vi "Run.vi"(8 "error in (no error)":errorcluster, 11 "LINX in":refnum<class "LINX.lvclass">) -> (0 "error out":errorcluster, 3 "LINX out":refnum<class "LINX.lvclass">)   [LabVIEW 2019, in "LINX.lvlib" / "LINX.lvclass"]
doc: "<b>Execution System:</b> Data Acquisition"
uses:
  LINX.lvclass
  <vilib>/MakerHub/LINX/Public/Peripherals/Analog/Analog Read N Chans.vi
  <vilib>/MakerHub/LINX/Public/Peripherals/Digital/Digital Read N Chans.vi
  <vilib>/MakerHub/LINX/Private/Local IO/LinxAnalogRead.vi
  <vilib>/MakerHub/LINX/Public/Utilities/Check Channel.vi
  <vilib>/MakerHub/LINX/Private/Local IO/LinxDigitalRead.vi
  <vilib>/MakerHub/LINX/Public/Utilities/Open Serial.vi
  <vilib>/MakerHub/LINX/Private/Utilties/Generate Error.vi
  Packed Libraries/Messaging.lvlibp/Send.vi
  Plugin Interfaces/Controller Interface/Controller Interface.lvlibp/Controller Interface Class/Controller Interface.lvclass
  <vilib>/MakerHub/LINX/LMH-LINX.lvlib
  C:/github/dataflowg/dataflow-dj/src/Plugin Interfaces/Controller Interface/Controller Interface.lvlibp/Controller Interface Class/Controller Interface.lvclass
panel:
  out "Error":errorcluster
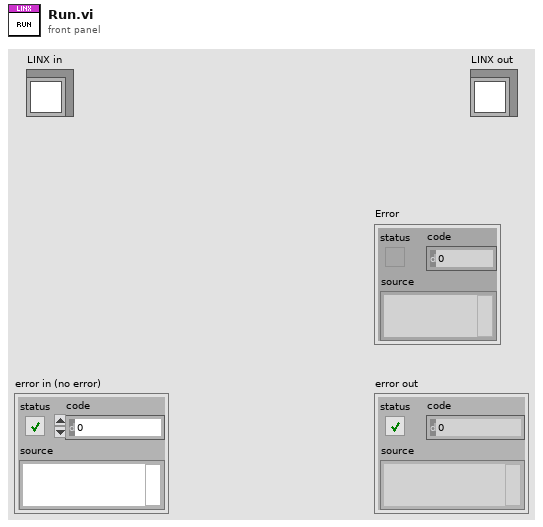
[diagram p1: front panel]
types:
  T1 = typedef "LINX.lvlib/LINX.lvclass/LINX Control Shortcut.ctl" = cluster{"Channel Type":T2, "Channel Number":u8, "Message Queue":string, "Event":string, "Target":string, "Momentary":bool, "Data":variant}
  T2 = typedef "LINX.lvlib/LINX.lvclass/LINX Channel Type.ctl" = enum16{"DI", "AI"}
  T3 = cluster{"value":string, "value":i32, T1[], T1[]}[]
  T4 = typedef "LMH-LINX.lvlib/LINX Ref.ctl" = cluster{"IO":T5, "Interface":T6, "LINX Device Config":T7}
  T5 = typedef "LMH-LINX.lvlib/Platform.ctl" = enum16{"Remote", "Local"}
  T6 = typedef "LMH-LINX.lvlib/Interface.ctl" = enum16{"Serial", "TCP"}
  T7 = typedef "LMH-LINX.lvlib/Device.lvlib/LINX Device Config.ctl" = cluster{"Interface":T6, "COM Port":refnum<visa-resource-name>, "TCP Configuration":T8, "Device Family":u8, "Device ID":u8, "Device Name":string, "TCP Ref":refnum<k5>, "Channels":T9}
  T8 = typedef "LMH-LINX.lvlib/Device.lvlib/TCP Config.ctl" = cluster{"IP Address":string, "Port":u16}
  T9 = typedef "LMH-LINX.lvlib/Channels.ctl" = cluster{"DI":u8[], "DO":u8[], "AI":u8[], "AO":u8[], "PWM":u8[], "QE":u8[], "UART":u8[], "I2C 2":u8[], "SPI":u8[], "CAN":u8[], "Servo":u8[], "AI Ref (V)":dbl, "AI Resolution (Bits)":u8, "AO Ref (V)":dbl, "AO Resolution (Bits)":u8}
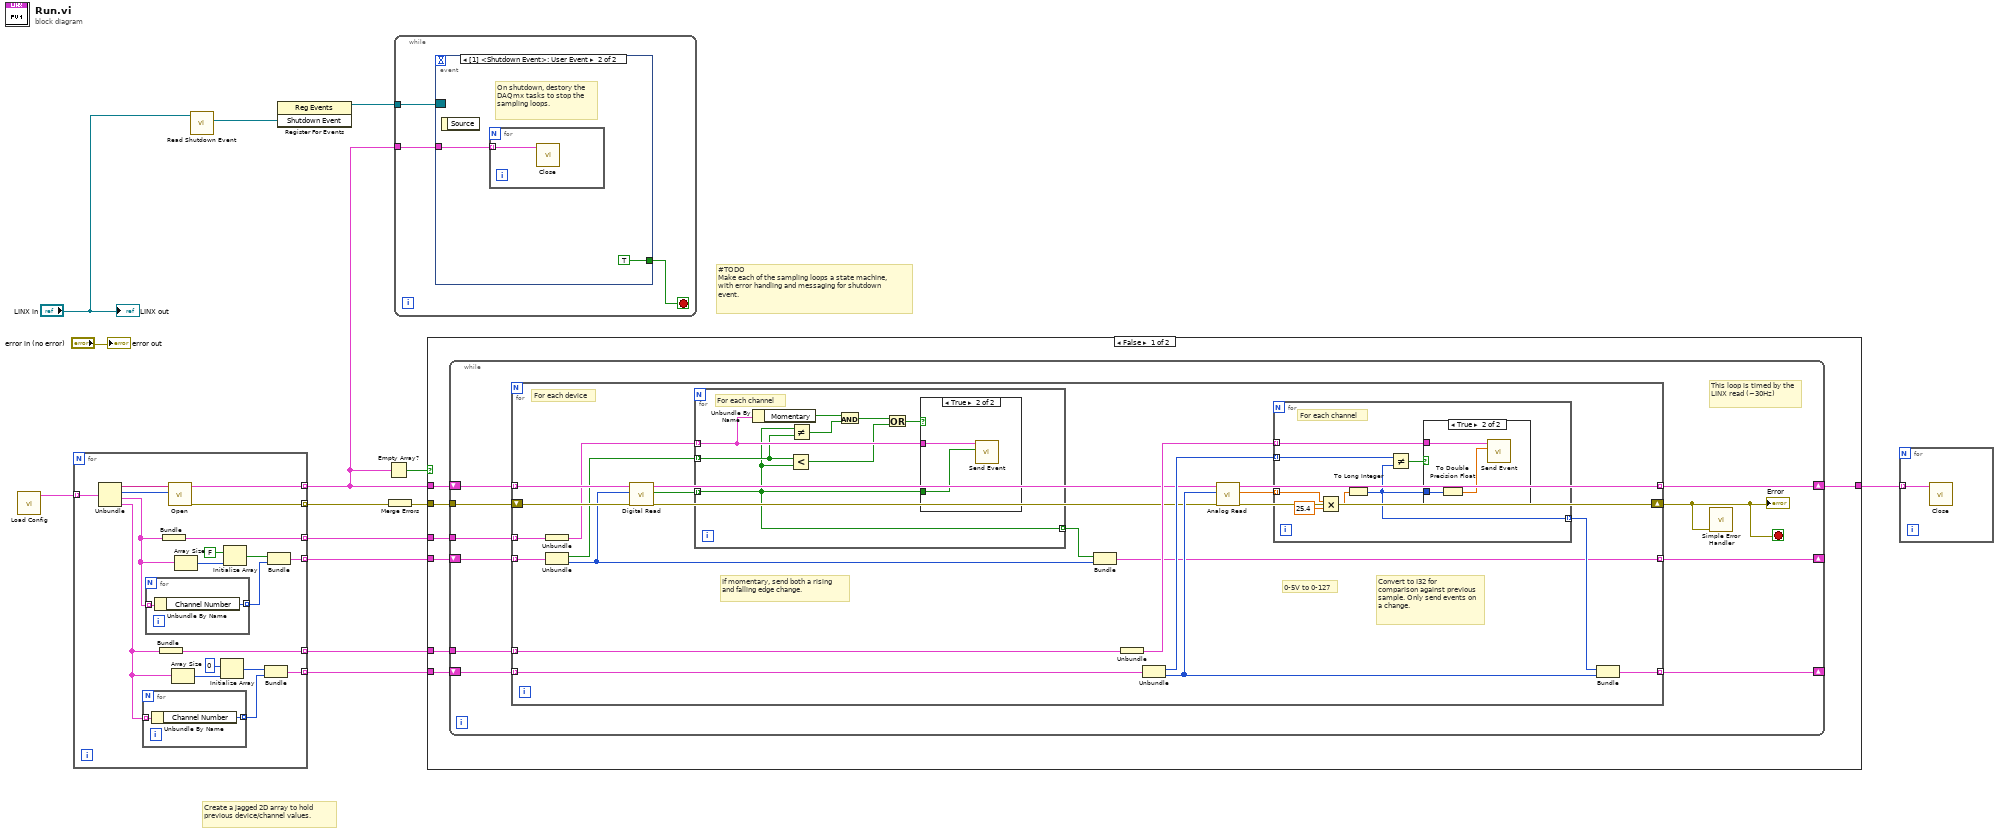
[diagram p0: block diagram]
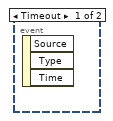
[diagram p5: hidden frame]
diagram:
  # "#TODO\nMake each of the sampling loops a state machine, with error handling and messaging for shutdown event."
  # "Create a jagged 2D array to hold previous device/channel values."
  n1 = call "Load Config.vi"() -> ("Array"=w4:T3)  [unwired: 10 in, 1 out]
  n2 = for {
    tunnel: [w28] -> w14 mode=indexing
    tunnel: [w33] -> w13 mode=indexing
    tunnel: [w29] -> w9 mode=indexing
    tunnel: [w23] -> w11 mode=indexing
    tunnel: w4 -> [w26] mode=indexing
    tunnel: [w16] -> w3 mode=indexing
    tunnel: [w15] -> w2 mode=indexing
    n3 = Unbundle(w26) -> ("value"=w25:string, "value"=w24:i32, w18:T1[], w22:T1[])
    n4 = for {
      tunnel: w22 -> [w37] mode=indexing
      tunnel: [w36] -> w27 mode=indexing
      n5 = Unbundle By Name(w37) -> ("Channel Number"=w36:u8)
    }
    n6 = for {
      tunnel: w18 -> [w35] mode=indexing
      tunnel: [w34] -> w21 mode=indexing
      n7 = Unbundle By Name(w35) -> ("Channel Number"=w34:u8)
    }
    n8 = Bundle(w22) -> (w23:cluster{T1[]})  [unwired: 1 in]
    n9 = Bundle(w18) -> (w16:cluster{T1[]})  [unwired: 1 in]
    n10 = call-poly <vilib>:"Open.vi"("Baud Rate Override"=w24, "Serial Port"=w25) -> ("Error Out"=w28:errorcluster, "LINX Resource"=w29:T4)  [unwired: 7 in, 1 out]
    n11 = Array Size(array=w22) -> (size(s)=w31:i32)
    n12 = Array Size(array=w18) -> (size(s)=w19:i32)
    n13 = Initialize Array(0 ("element"), w31) -> (w30:i32[])
    n14 = Initialize Array(FALSE, w19) -> (w20:bool[])
    n15 = Bundle(w30, w27) -> (w33:cluster{i32[], u8[]})  [unwired: 1 in]
    n16 = Bundle(w20, w21) -> (w15:cluster{bool[], u8[]})  [unwired: 1 in]
  }
  n17 = call "Read Shutdown Event.vi"("Controller Interface in"="LINX in") -> ("Shutdown Event"=w5:refnum<user-event>)  [unwired: 9 in, 1 out]
  n18 = register-events(w5) -> (reference out=w12:refnum<event-registration>)  [unwired: 2 in, 1 out]
  n19 = Empty Array?(array=w9) -> (empty?=w8:bool)
  n20 = Merge Errors(w14) -> (w10:errorcluster)
  n21 = while {
    tunnel: w12 -> [w40]
    tunnel: w9 -> [w38]
    stop <- w39 stop-if-true
    n22 = event shown="[1] <Shutdown Event>: User Event" {
      selector: w40 -> [_ _]
      dyn-events: _ -> [_ _]
      timeout: _ -> [_ _]
      tunnel: [_ TRUE] -> w39
      tunnel: w38 -> [_ w41]
      event Timeout {
        n23 = event-data() -> ()  [unwired: 1 in, 3 out]
      }
      event User Event {
        # "On shutdown, destory the DAQmx tasks to stop the sampling loops."
        n24 = event-data() -> ()  [unwired: 1 in, 1 out]
        n25 = for {
          tunnel: w41 -> [w43] mode=indexing
          n26 = call <vilib>:"Close.vi"("LINX Resource"=w43) -> ()  [unwired: 10 in, 1 out]
        }
      }
    }
  }
  n27 = case shown="False" w8 {
    tunnel: w13 -> [w50 _]
    tunnel: w11 -> [w49 _]
    tunnel: w10 -> [w48 _]
    tunnel: w9 -> [w47 w103]
    tunnel: w3 -> [w46 _]
    tunnel: w2 -> [w45 _]
    tunnel: [w44 w103] -> w1
    frame False {
      n28 = while {
        tunnel: w48 -> [w59]
        tunnel: w49 -> [w57]
        shift-right: [w56] -> _
        shift-left: w50 -> [w58]
        shift-right: [w55] -> w44
        shift-left: w47 -> [w60]
        tunnel: w46 -> [w53]
        shift-right: [w51] -> _
        shift-left: w45 -> [w52]
        stop <- w54 stop-if-true
        # "This loop is timed by the LINX read (~30Hz)"
        n29 = for {
          tunnel: w60 -> [w69] mode=indexing
          tunnel: w58 -> [w79] mode=indexing
          tunnel: w57 -> [w82] mode=indexing
          tunnel: [w77] -> w56 mode=indexing
          shift-right: [w76] -> w54
          shift-left: w59 -> [w68]
          tunnel: [w74] -> w55 mode=indexing
          tunnel: w53 -> [w72] mode=indexing
          tunnel: w52 -> [w71] mode=indexing
          tunnel: [w61] -> w51 mode=indexing
          # "0-5V to 0-127"
          # "Convert to I32 for comparison against previous sample. Only send events on a change."
          # "If momentary, send both a rising and falling edge change."
          # "For each device"
          n30 = Unbundle(w72) -> (w65:T1[])
          n31 = Unbundle(w71) -> (w64:bool[], w63:u8[])
          n32 = call-poly <vilib>:"Digital Read.vi"("Error In"=w68, "DI Channels"=w63, "LINX Resource"=w69) -> ("Error Out"=w67:errorcluster, "Values"=w66:bool[], "LINX Resource"=w70:T4)  [unwired: 6 in]
          n33 = for {
            tunnel: w66 -> [w85] mode=indexing
            tunnel: w65 -> [w89] mode=indexing
            tunnel: w64 -> [w86] mode=indexing
            tunnel: [w85] -> w62 mode=indexing
            # "For each channel"
            n34 = Unbundle By Name(w89) -> ("Momentary"=w88:bool)
            n35 = Less?(x=w86, y=w85) -> (x < y?=w84:bool)
            n36 = Not Equal?(x=w85, y=w86) -> (x != y?=w90:bool)
            n37 = And(x=w88, y=w90) -> (x .and. y?=w87:bool)
            n38 = Or(x=w87, y=w84) -> (x .or. y?=w83:bool)
            n39 = case shown="True" w83 {
              tunnel: w89 -> [_ w92]
              tunnel: w85 -> [_ w91]
              frame False {
              }
              frame True {
                n40 = call "Send Event.vi"("Data"=w91, "LINX Shortcut"=w92) -> ()  [unwired: 10 in]
              }
            }
          }
          n41 = Bundle(w62, w63) -> (w61:cluster{bool[], u8[]})  [unwired: 1 in]
          n42 = Unbundle(w82) -> (w78:T1[])
          n43 = Unbundle(w79) -> (w80:i32[], w73:u8[])
          n44 = call-poly <vilib>:"Analog Read.vi"("Error In"=w67, "AI Channel(s)"=w73, "LINX Resource"=w70) -> ("Error Out"=w76:errorcluster, "Voltages"=w75:dbl[], "LINX Resource"=w74:T4)  [unwired: 5 in, 1 out]
          n45 = for {
            tunnel: w75 -> [w94] mode=indexing
            tunnel: w80 -> [w99] mode=indexing
            tunnel: w78 -> [w98] mode=indexing
            tunnel: [w96] -> w81 mode=indexing
            # "For each channel"
            n46 = Multiply(x=w94, y=25.4) -> (x*y=w95:dbl)
            n47 = To Long Integer(number=w95) -> (32bit integer=w96:i32)
            n48 = Not Equal?(x=w99, y=w96) -> (x != y?=w97:bool)
            n49 = case shown="True" w97 {
              tunnel: w98 -> [_ w101]
              tunnel: w96 -> [_ w102]
              frame False {
              }
              frame True {
                n50 = To Double Precision Float(number=w102) -> (double precision float=w100:dbl)
                n51 = call "Send Event.vi"("Data"=w100, "LINX Shortcut"=w101) -> ()  [unwired: 10 in]
              }
            }
          }
          n52 = Bundle(w81, w73) -> (w77:cluster{i32[], u8[]})  [unwired: 1 in]
        }
        "Error" <- w54
        n53 = call <vilib>:"Simple Error Handler.vi"("error in (no error)"=w54) -> ()  [unwired: 4 in, 5 out]
      }
    }
    frame True {
    }
  }
  n54 = for {
    tunnel: w1 -> [w104] mode=indexing
    n55 = call <vilib>:"Close.vi"("LINX Resource"=w104) -> ()  [unwired: 10 in, 1 out]
  }
  "error out" <- "error in (no error)"
  "LINX out" <- "LINX in"
